vi "Disconnect source-meter(SubIV).vi"(8 "Error In":errorcluster, 11 "Loop data In":T1={"Persistent"={"Last file"=path "", "Last user"="", "Users"=[]}, "Temp handle"={"Connected"=FALSE, "Temp ctrl"={"Gain (P)"=0.0, "Reset (I)"=0.0, "Rate (D)"=0.0, "Stabilization rate"=0.0, "Stabilization delta"=0.0, "Type"=enum."Lake Shore 325", "Custom temp ctrl"={"VISA resource name"=""}, "Lakeshore 325"={"VISA name"="", "Loop"=0, "Heater Range"=1, "Heater Resistance"=0, "Sample sensor"=0, "Fast sensor"=0, "Slow sensor"=0}, "Lakeshore 331"={"VISA name"="", "Loop"=1, "Heater Range"=0, "Sample sensor"=0, "Fast sensor"=0, "Slow sensor"=0}, "Lakeshore 332"={"VISA name"="", "Loop"=1, "Heater Range"=0, "Sample sensor"=0, "Fast sensor"=0, "Slow sensor"=0}, "Lakeshore 335"={"VISA name"="", "Loop"=1, "Sample sensor"=0, "Fast sensor"=0, "Slow sensor"=0}}}, "Paths"={"Manual"=path "", "Settings"=path "", "Persistent"=path "", "Work dir."=path ""}, "Settings"={"MFIA"={"Address"="", "Use compensation"=TRUE, "Shut down gracefully"=FALSE}, "Temp ctrl"={"Gain (P)"=0.0, "Reset (I)"=0.0, "Rate (D)"=0.0, "Stabilization rate"=0.0, "Stabilization delta"=0.0, "Type"=enum."Lake Shore 325", "Custom temp ctrl"={"VISA resource name"=""}, "Lakeshore 325"={"VISA name"="", "Loop"=0, "Heater Range"=1, "Heater Resistance"=0, "Sample sensor"=0, "Fast sensor"=0, "Slow sensor"=0}, "Lakeshore 331"={"VISA name"="", "Loop"=1, "Heater Range"=0, "Sample sensor"=0, "Fast sensor"=0, "Slow sensor"=0}, "Lakeshore 332"={"VISA name"="", "Loop"=1, "Heater Range"=0, "Sample sensor"=0, "Fast sensor"=0, "Slow sensor"=0}, "Lakeshore 335"={"VISA name"="", "Loop"=1, "Sample sensor"=0, "Fast sensor"=0, "Slow sensor"=0}}, "Source-meter"={"Type"=enum."Custom", "Custom source-meter"={"VISA resource name"=""}, "Keithley 2600"={"VISA name"=""}}, "Other"={"Enable OriginLab"=FALSE, "Reader mode"=FALSE, "Auto-save"=FALSE}, "Defaults"={"IV properties"={"T"=0.0, "Vstart"=-0.5, "Vstop"=0.5, "Vpoints"=10.0, "Settling"=0.01, "I limit"=0.1, "Log mapping"=FALSE, "Averaging"=0.0}, "CV properties"={"T"=0.0, "Vstart"=-0.5, "Vstop"=0.5, "Vpoints"=10.0, "Precision"=enum."Normal", "Test signal"=0.01, "Auto I range"=FALSE, "Test frequency"=100000.0, "I range"=-2.0, "V range"=10.0, "Log mapping"=FALSE, "Rel perm"=0.0, "Area"=0.0}, "DLTS properties"={"Tstart"=0.0, "Instant start"=FALSE, "Tstop"=0.0, "T rate"=0.0, "Test signal"=0.0, "Test frequency"=0.0, "Bandwidth"=0.0, "Averaging"=0.0, "Vbias"=0.0, "Vpulse"=0.0, "pulse length"=0.0, "Pulse 2"=FALSE, "Vpulse 2"=0.0, "pulse length 2"=0.0, "I range"=-2.0, "V range"=10.0, "Emission rate"=[], "Sampling rate"=0.0, "Acq. delay"=0.0}, "LDLTS properties"={"T"=0.0, "Test signal"=0.0, "Test frequency"=0.0, "Bandwidth"=0.0, "Averaging"=0.0, "Vbias"=0.0, "Vpulse"=0.0, "pulse length"=0.0, "Pulse 2"=FALSE, "Vpulse 2"=0.0, "pulse length 2"=0.0, "I range"=-2.0, "V range"=10.0, "Sampling rate"=0.0, "Acq. delay"=0.0, "Sampling time"=0.0}}}, "Software version"=0.0, "MFIA handle"={"ziHandle"={"handleValid"=FALSE, "Conn"=0, "Path Prefix"="", "Handle"=0, "Connected"=FALSE, "Clockbase(s)"=0.0}, "Selected device"="", "ziModHandle"={"handleValid"=FALSE, "Conn"=0, "ModHandle"=0, "moduleID"="", "Path Prefix"=""}}, "Source-meter handle"={"Connected"=FALSE, "Source-meter"={"Type"=enum."Custom", "Custom source-meter"={"VISA resource name"=""}, "Keithley 2600"={"VISA name"=""}}}} {"MFIA handle"."ziModHandle"."ModHandle" format="0x%08x"; "MFIA handle"."ziModHandle"."Conn" format="0x%08x"; "MFIA handle"."ziHandle"."Handle" format="0x%08x"; "MFIA handle"."ziHandle"."Conn" format="0x%08x"; "Settings"."Defaults"."LDLTS properties"."V range" items=["10mV"=0.01, "100mV"=0.1, "1V"=1.0, "10V"=10.0]; "Settings"."Defaults"."LDLTS properties"."I range" items=["100nA"=-7.0, "1µA"=-6.0, "10µA"=-5.0, "100µA"=-4.0, "1mA"=-3.0, "10mA"=-2.0]; "Settings"."Defaults"."DLTS properties"."V range" items=["10mV"=0.01, "100mV"=0.1, "1V"=1.0, "10V"=10.0]; "Settings"."Defaults"."DLTS properties"."I range" items=["10mV"=0.01, "100mV"=0.1, "1V"=1.0, "10V"=10.0]; "Settings"."Defaults"."CV properties"."V range" items=["10mV"=0.01, "100mV"=0.1, "1V"=1.0, "10V"=10.0]; "Settings"."Defaults"."CV properties"."I range" items=["100nA"=-7.0, "1µA"=-6.0, "10µA"=-5.0, "100µA"=-4.0, "1mA"=-3.0, "10mA"=-2.0]; "Settings"."Defaults"."IV properties"."Settling" min=0.0 max=65535.0; "Settings"."Temp ctrl"."Lakeshore 335"."Slow sensor" items=["A", "B"]; "Settings"."Temp ctrl"."Lakeshore 335"."Fast sensor" items=["A", "B"]; "Settings"."Temp ctrl"."Lakeshore 335"."Sample sensor" items=["A", "B"]; "Settings"."Temp ctrl"."Lakeshore 335"."Loop" items=["Loop 1"=1, "Loop 2"=2]; "Settings"."Temp ctrl"."Lakeshore 332"."Slow sensor" items=["A", "B"]; "Settings"."Temp ctrl"."Lakeshore 332"."Fast sensor" items=["A", "B"]; "Settings"."Temp ctrl"."Lakeshore 332"."Sample sensor" items=["A", "B"]; "Settings"."Temp ctrl"."Lakeshore 332"."Heater Range" items=["Off", "Low (0.5W)", "Med (5W)", "High (50W)"]; "Settings"."Temp ctrl"."Lakeshore 332"."Loop" items=["Loop 1", "Loop 2"]; "Settings"."Temp ctrl"."Lakeshore 331"."Slow sensor" items=["A", "B"]; "Settings"."Temp ctrl"."Lakeshore 331"."Fast sensor" items=["A", "B"]; "Settings"."Temp ctrl"."Lakeshore 331"."Sample sensor" items=["A", "B"]; "Settings"."Temp ctrl"."Lakeshore 331"."Heater Range" items=["Off", "Low (0.5W)", "Med (5W)", "High (50W)"]; "Settings"."Temp ctrl"."Lakeshore 331"."Loop" items=["Loop 1", "Loop 2"]; "Settings"."Temp ctrl"."Lakeshore 325"."Slow sensor" items=["A", "B"]; "Settings"."Temp ctrl"."Lakeshore 325"."Fast sensor" items=["A", "B"]; "Settings"."Temp ctrl"."Lakeshore 325"."Sample sensor" items=["A", "B"]; "Settings"."Temp ctrl"."Lakeshore 325"."Heater Resistance" items=["25 Ohm"=1, "50 Ohm"=2]; "Settings"."Temp ctrl"."Lakeshore 325"."Heater Range" items=["Off", "Low (loop 1) or On (loop 2)", "High (loop 1)"]; "Settings"."Temp ctrl"."Lakeshore 325"."Loop" items=["Loop 1"=1, "Loop 2"=2]; "Temp handle"."Temp ctrl"."Lakeshore 335"."Slow sensor" items=["A", "B"]; "Temp handle"."Temp ctrl"."Lakeshore 335"."Fast sensor" items=["A", "B"]; "Temp handle"."Temp ctrl"."Lakeshore 335"."Sample sensor" items=["A", "B"]; "Temp handle"."Temp ctrl"."Lakeshore 335"."Loop" items=["Loop 1"=1, "Loop 2"=2]; "Temp handle"."Temp ctrl"."Lakeshore 332"."Slow sensor" items=["A", "B"]; "Temp handle"."Temp ctrl"."Lakeshore 332"."Fast sensor" items=["A", "B"]; "Temp handle"."Temp ctrl"."Lakeshore 332"."Sample sensor" items=["A", "B"]; "Temp handle"."Temp ctrl"."Lakeshore 332"."Heater Range" items=["Off", "Low (0.5W)", "Med (5W)", "High (50W)"]; "Temp handle"."Temp ctrl"."Lakeshore 332"."Loop" items=["Loop 1", "Loop 2"]; "Temp handle"."Temp ctrl"."Lakeshore 331"."Slow sensor" items=["A", "B"]; "Temp handle"."Temp ctrl"."Lakeshore 331"."Fast sensor" items=["A", "B"]; "Temp handle"."Temp ctrl"."Lakeshore 331"."Sample sensor" items=["A", "B"]; "Temp handle"."Temp ctrl"."Lakeshore 331"."Heater Range" items=["Off", "Low (0.5W)", "Med (5W)", "High (50W)"]; "Temp handle"."Temp ctrl"."Lakeshore 331"."Loop" items=["Loop 1", "Loop 2"]; "Temp handle"."Temp ctrl"."Lakeshore 325"."Slow sensor" items=["A", "B"]; "Temp handle"."Temp ctrl"."Lakeshore 325"."Fast sensor" items=["A", "B"]; "Temp handle"."Temp ctrl"."Lakeshore 325"."Sample sensor" items=["A", "B"]; "Temp handle"."Temp ctrl"."Lakeshore 325"."Heater Resistance" items=["25 Ohm"=1, "50 Ohm"=2]; "Temp handle"."Temp ctrl"."Lakeshore 325"."Heater Range" items=["Off", "Low (loop 1) or On (loop 2)", "High (loop 1)"]; "Temp handle"."Temp ctrl"."Lakeshore 325"."Loop" items=["Loop 1"=1, "Loop 2"=2]}) -> (0 "Error Out":errorcluster, 3 "Loop data Out":T1={"Persistent"={"Last file"=path "", "Last user"="", "Users"=[]}, "Temp handle"={"Connected"=FALSE, "Temp ctrl"={"Gain (P)"=0.0, "Reset (I)"=0.0, "Rate (D)"=0.0, "Stabilization rate"=0.0, "Stabilization delta"=0.0, "Type"=enum."Lake Shore 325", "Custom temp ctrl"={"VISA resource name"=""}, "Lakeshore 325"={"VISA name"="", "Loop"=0, "Heater Range"=1, "Heater Resistance"=0, "Sample sensor"=0, "Fast sensor"=0, "Slow sensor"=0}, "Lakeshore 331"={"VISA name"="", "Loop"=1, "Heater Range"=0, "Sample sensor"=0, "Fast sensor"=0, "Slow sensor"=0}, "Lakeshore 332"={"VISA name"="", "Loop"=1, "Heater Range"=0, "Sample sensor"=0, "Fast sensor"=0, "Slow sensor"=0}, "Lakeshore 335"={"VISA name"="", "Loop"=1, "Sample sensor"=0, "Fast sensor"=0, "Slow sensor"=0}}}, "Paths"={"Manual"=path "", "Settings"=path "", "Persistent"=path "", "Work dir."=path ""}, "Settings"={"MFIA"={"Address"="", "Use compensation"=TRUE, "Shut down gracefully"=FALSE}, "Temp ctrl"={"Gain (P)"=0.0, "Reset (I)"=0.0, "Rate (D)"=0.0, "Stabilization rate"=0.0, "Stabilization delta"=0.0, "Type"=enum."Lake Shore 325", "Custom temp ctrl"={"VISA resource name"=""}, "Lakeshore 325"={"VISA name"="", "Loop"=0, "Heater Range"=1, "Heater Resistance"=0, "Sample sensor"=0, "Fast sensor"=0, "Slow sensor"=0}, "Lakeshore 331"={"VISA name"="", "Loop"=1, "Heater Range"=0, "Sample sensor"=0, "Fast sensor"=0, "Slow sensor"=0}, "Lakeshore 332"={"VISA name"="", "Loop"=1, "Heater Range"=0, "Sample sensor"=0, "Fast sensor"=0, "Slow sensor"=0}, "Lakeshore 335"={"VISA name"="", "Loop"=1, "Sample sensor"=0, "Fast sensor"=0, "Slow sensor"=0}}, "Source-meter"={"Type"=enum."Custom", "Custom source-meter"={"VISA resource name"=""}, "Keithley 2600"={"VISA name"=""}}, "Other"={"Enable OriginLab"=FALSE, "Reader mode"=FALSE, "Auto-save"=FALSE}, "Defaults"={"IV properties"={"T"=0.0, "Vstart"=-0.5, "Vstop"=0.5, "Vpoints"=10.0, "Settling"=0.01, "I limit"=0.1, "Log mapping"=FALSE, "Averaging"=0.0}, "CV properties"={"T"=0.0, "Vstart"=-0.5, "Vstop"=0.5, "Vpoints"=10.0, "Precision"=enum."Normal", "Test signal"=0.01, "Auto I range"=FALSE, "Test frequency"=100000.0, "I range"=-2.0, "V range"=10.0, "Log mapping"=FALSE, "Rel perm"=0.0, "Area"=0.0}, "DLTS properties"={"Tstart"=0.0, "Instant start"=FALSE, "Tstop"=0.0, "T rate"=0.0, "Test signal"=0.0, "Test frequency"=0.0, "Bandwidth"=0.0, "Averaging"=0.0, "Vbias"=0.0, "Vpulse"=0.0, "pulse length"=0.0, "Pulse 2"=FALSE, "Vpulse 2"=0.0, "pulse length 2"=0.0, "I range"=-2.0, "V range"=10.0, "Emission rate"=[], "Sampling rate"=0.0, "Acq. delay"=0.0}, "LDLTS properties"={"T"=0.0, "Test signal"=0.0, "Test frequency"=0.0, "Bandwidth"=0.0, "Averaging"=0.0, "Vbias"=0.0, "Vpulse"=0.0, "pulse length"=0.0, "Pulse 2"=FALSE, "Vpulse 2"=0.0, "pulse length 2"=0.0, "I range"=-2.0, "V range"=10.0, "Sampling rate"=0.0, "Acq. delay"=0.0, "Sampling time"=0.0}}}, "Software version"=0.0, "MFIA handle"={"ziHandle"={"handleValid"=FALSE, "Conn"=0, "Path Prefix"="", "Handle"=0, "Connected"=FALSE, "Clockbase(s)"=0.0}, "Selected device"="", "ziModHandle"={"handleValid"=FALSE, "Conn"=0, "ModHandle"=0, "moduleID"="", "Path Prefix"=""}}, "Source-meter handle"={"Connected"=FALSE, "Source-meter"={"Type"=enum."Custom", "Custom source-meter"={"VISA resource name"=""}, "Keithley 2600"={"VISA name"=""}}}} {"MFIA handle"."ziModHandle"."ModHandle" format="0x%08x"; "MFIA handle"."ziModHandle"."Conn" format="0x%08x"; "MFIA handle"."ziHandle"."Handle" format="0x%08x"; "MFIA handle"."ziHandle"."Conn" format="0x%08x"; "Settings"."Defaults"."LDLTS properties"."V range" items=["10mV"=0.01, "100mV"=0.1, "1V"=1.0, "10V"=10.0]; "Settings"."Defaults"."LDLTS properties"."I range" items=["100nA"=-7.0, "1µA"=-6.0, "10µA"=-5.0, "100µA"=-4.0, "1mA"=-3.0, "10mA"=-2.0]; "Settings"."Defaults"."DLTS properties"."V range" items=["10mV"=0.01, "100mV"=0.1, "1V"=1.0, "10V"=10.0]; "Settings"."Defaults"."DLTS properties"."I range" items=["10mV"=0.01, "100mV"=0.1, "1V"=1.0, "10V"=10.0]; "Settings"."Defaults"."CV properties"."V range" items=["10mV"=0.01, "100mV"=0.1, "1V"=1.0, "10V"=10.0]; "Settings"."Defaults"."CV properties"."I range" items=["100nA"=-7.0, "1µA"=-6.0, "10µA"=-5.0, "100µA"=-4.0, "1mA"=-3.0, "10mA"=-2.0]; "Settings"."Defaults"."IV properties"."Settling" min=0.0 max=65535.0; "Settings"."Temp ctrl"."Lakeshore 335"."Slow sensor" items=["A", "B"]; "Settings"."Temp ctrl"."Lakeshore 335"."Fast sensor" items=["A", "B"]; "Settings"."Temp ctrl"."Lakeshore 335"."Sample sensor" items=["A", "B"]; "Settings"."Temp ctrl"."Lakeshore 335"."Loop" items=["Loop 1"=1, "Loop 2"=2]; "Settings"."Temp ctrl"."Lakeshore 332"."Slow sensor" items=["A", "B"]; "Settings"."Temp ctrl"."Lakeshore 332"."Fast sensor" items=["A", "B"]; "Settings"."Temp ctrl"."Lakeshore 332"."Sample sensor" items=["A", "B"]; "Settings"."Temp ctrl"."Lakeshore 332"."Heater Range" items=["Off", "Low (0.5W)", "Med (5W)", "High (50W)"]; "Settings"."Temp ctrl"."Lakeshore 332"."Loop" items=["Loop 1", "Loop 2"]; "Settings"."Temp ctrl"."Lakeshore 331"."Slow sensor" items=["A", "B"]; "Settings"."Temp ctrl"."Lakeshore 331"."Fast sensor" items=["A", "B"]; "Settings"."Temp ctrl"."Lakeshore 331"."Sample sensor" items=["A", "B"]; "Settings"."Temp ctrl"."Lakeshore 331"."Heater Range" items=["Off", "Low (0.5W)", "Med (5W)", "High (50W)"]; "Settings"."Temp ctrl"."Lakeshore 331"."Loop" items=["Loop 1", "Loop 2"]; "Settings"."Temp ctrl"."Lakeshore 325"."Slow sensor" items=["A", "B"]; "Settings"."Temp ctrl"."Lakeshore 325"."Fast sensor" items=["A", "B"]; "Settings"."Temp ctrl"."Lakeshore 325"."Sample sensor" items=["A", "B"]; "Settings"."Temp ctrl"."Lakeshore 325"."Heater Resistance" items=["25 Ohm"=1, "50 Ohm"=2]; "Settings"."Temp ctrl"."Lakeshore 325"."Heater Range" items=["Off", "Low (loop 1) or On (loop 2)", "High (loop 1)"]; "Settings"."Temp ctrl"."Lakeshore 325"."Loop" items=["Loop 1"=1, "Loop 2"=2]; "Temp handle"."Temp ctrl"."Lakeshore 335"."Slow sensor" items=["A", "B"]; "Temp handle"."Temp ctrl"."Lakeshore 335"."Fast sensor" items=["A", "B"]; "Temp handle"."Temp ctrl"."Lakeshore 335"."Sample sensor" items=["A", "B"]; "Temp handle"."Temp ctrl"."Lakeshore 335"."Loop" items=["Loop 1"=1, "Loop 2"=2]; "Temp handle"."Temp ctrl"."Lakeshore 332"."Slow sensor" items=["A", "B"]; "Temp handle"."Temp ctrl"."Lakeshore 332"."Fast sensor" items=["A", "B"]; "Temp handle"."Temp ctrl"."Lakeshore 332"."Sample sensor" items=["A", "B"]; "Temp handle"."Temp ctrl"."Lakeshore 332"."Heater Range" items=["Off", "Low (0.5W)", "Med (5W)", "High (50W)"]; "Temp handle"."Temp ctrl"."Lakeshore 332"."Loop" items=["Loop 1", "Loop 2"]; "Temp handle"."Temp ctrl"."Lakeshore 331"."Slow sensor" items=["A", "B"]; "Temp handle"."Temp ctrl"."Lakeshore 331"."Fast sensor" items=["A", "B"]; "Temp handle"."Temp ctrl"."Lakeshore 331"."Sample sensor" items=["A", "B"]; "Temp handle"."Temp ctrl"."Lakeshore 331"."Heater Range" items=["Off", "Low (0.5W)", "Med (5W)", "High (50W)"]; "Temp handle"."Temp ctrl"."Lakeshore 331"."Loop" items=["Loop 1", "Loop 2"]; "Temp handle"."Temp ctrl"."Lakeshore 325"."Slow sensor" items=["A", "B"]; "Temp handle"."Temp ctrl"."Lakeshore 325"."Fast sensor" items=["A", "B"]; "Temp handle"."Temp ctrl"."Lakeshore 325"."Sample sensor" items=["A", "B"]; "Temp handle"."Temp ctrl"."Lakeshore 325"."Heater Resistance" items=["25 Ohm"=1, "50 Ohm"=2]; "Temp handle"."Temp ctrl"."Lakeshore 325"."Heater Range" items=["Off", "Low (loop 1) or On (loop 2)", "High (loop 1)"]; "Temp handle"."Temp ctrl"."Lakeshore 325"."Loop" items=["Loop 1"=1, "Loop 2"=2]})   [LabVIEW 2019]
doc: "Terminates connection with source meter"
uses:
  Type defs/Loop data Type Def.ctl
  Type defs/Persistent Type Def.ctl
  Type defs/Temp handle Type Def.ctl
  Type defs/Temp ctrl Type Def.ctl
  Custom devices/Custom temp ctrl settings.ctl
  Type defs/Paths Type Def.ctl
  Type defs/Settings Type Def.ctl
  Type defs/Imps Type Def.ctl
  Type defs/Source-meter Type Def.ctl
  Custom devices/Custom source-meter settings.ctl
  Type defs/Other settings Type Def.ctl
  Type defs/IV properties Type Def.ctl
  Type defs/CV properties Type Def.ctl
  Type defs/DLTS properties Type Def.ctl
  Type defs/LDLTS properties Type Def.ctl
  Type defs/MFIA handle Type Def.ctl
  <instrlib>/Zurich Instruments LabOne/Public/ziTypeHandle.ctl
  <instrlib>/Zurich Instruments LabOne/Public/Modules/ziTypeModHandle.ctl
  Type defs/Source-meter handle Type Def.ctl
  <instrlib>/Keithley 2600 Series/Keithley 2600 Series.lvlib
  <instrlib>/Zurich Instruments LabOne/Zurich Instruments LabOne.lvlib
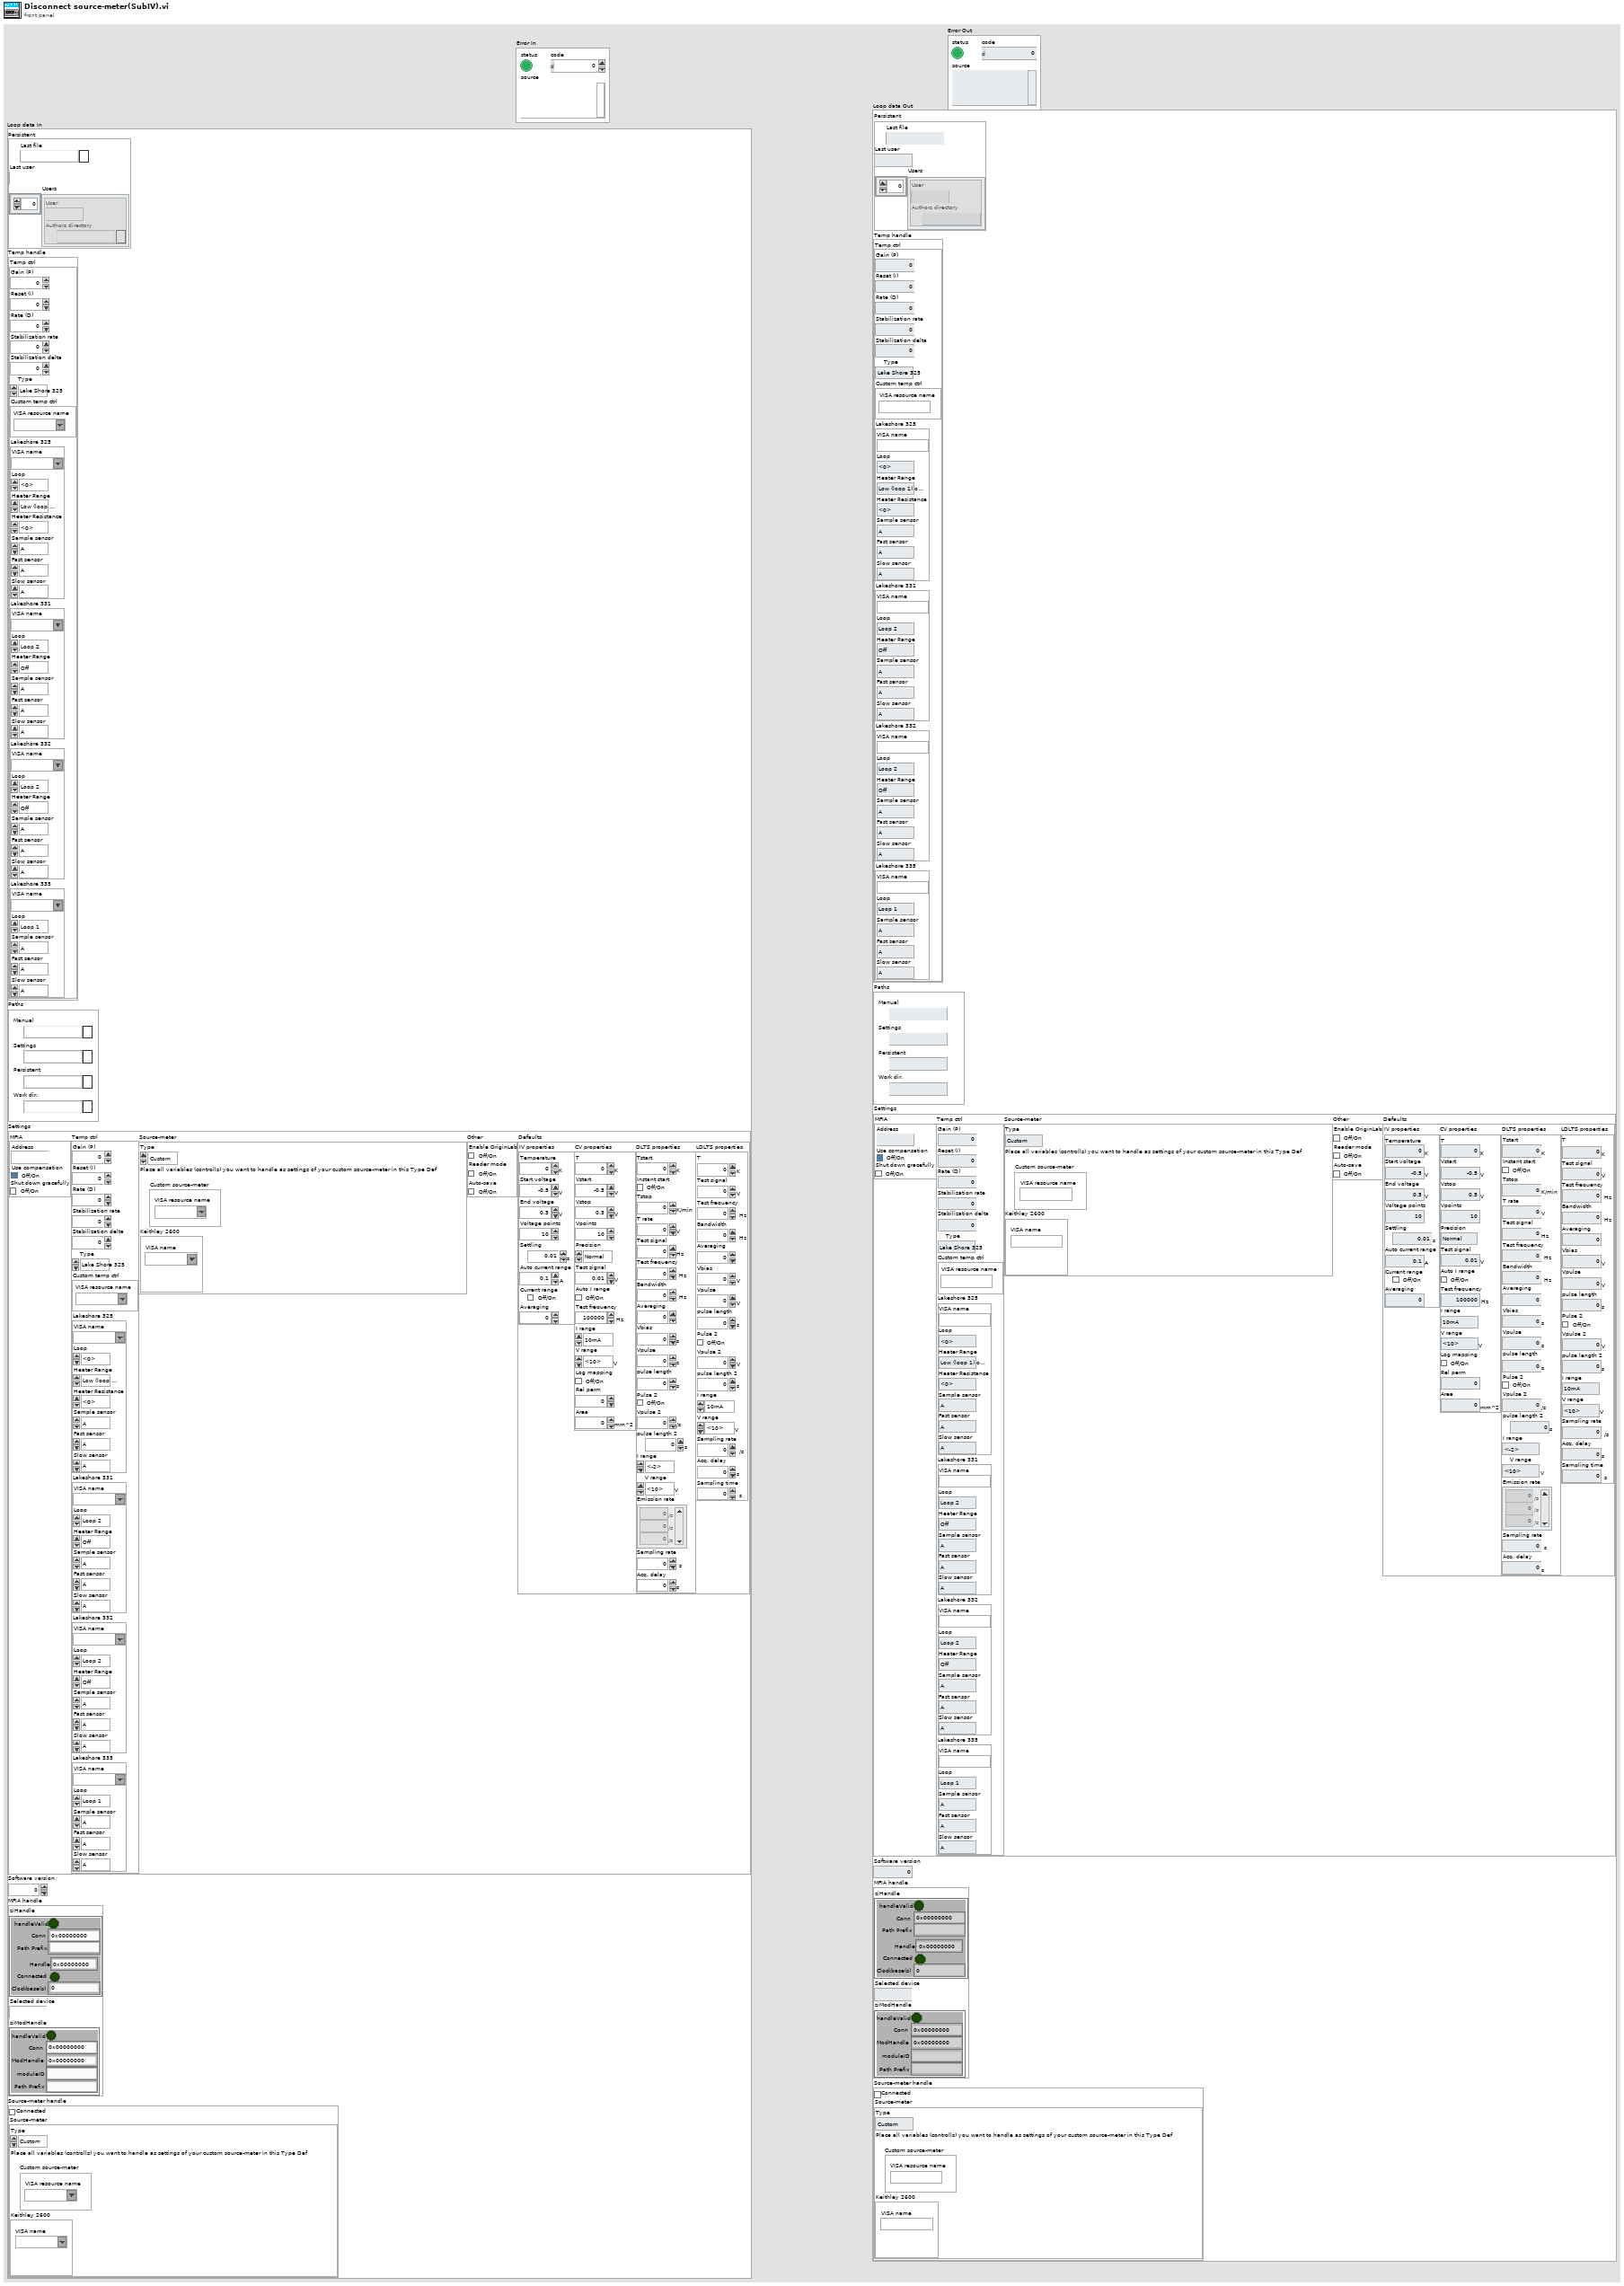
[diagram p1: front panel]
types:
  T1 = typedef "Loop data Type Def.ctl" = cluster{"Persistent":T2, "Temp handle":T3, "Paths":T6, "Settings":T7, "Software version":dbl, "MFIA handle":T16, "Source-meter handle":T19}
  T2 = typedef "Persistent Type Def.ctl" = cluster{"Last file":path, "Last user":string, "Users":cluster{"User":string, "Authors directory":path}[]}
  T3 = typedef "Temp handle Type Def.ctl" = cluster{"Connected":bool, "Temp ctrl":T4}
  T4 = typedef "Temp ctrl Type Def.ctl" = cluster{"Gain (P)":dbl, "Reset (I)":dbl, "Rate (D)":dbl, "Stabilization rate":dbl, "Stabilization delta":dbl, "Type":enum16{"Custom", "Lake Shore 325", "Lake Shore 331", "Lake Shore 332", "Lake Shore 335"}, "Custom temp ctrl":T5, "Lakeshore 325":cluster{"VISA name":refnum<visa-resource-name>, "Loop":u16, "Heater Range":u16, "Heater Resistance":u16, "Sample sensor":u16, "Fast sensor":u16, "Slow sensor":u16}, "Lakeshore 331":cluster{"VISA name":refnum<visa-resource-name>, "Loop":u16, "Heater Range":u16, "Sample sensor":u16, "Fast sensor":u16, "Slow sensor":u16}, "Lakeshore 332":cluster{"VISA name":refnum<visa-resource-name>, "Loop":u16, "Heater Range":u16, "Sample sensor":u16, "Fast sensor":u16, "Slow sensor":u16}, "Lakeshore 335":cluster{"VISA name":refnum<visa-resource-name>, "Loop":u16, "Sample sensor":u16, "Fast sensor":u16, "Slow sensor":u16}}
  T5 = typedef "Custom temp ctrl settings.ctl" = cluster{"VISA resource name":refnum<visa-resource-name>}
  T6 = typedef "Paths Type Def.ctl" = cluster{"Manual":path, "Settings":path, "Persistent":path, "Work dir.":path}
  T7 = typedef "Settings Type Def.ctl" = cluster{"MFIA":T8, "Temp ctrl":T4, "Source-meter":T9, "Other":T11, "Defaults":cluster{"IV properties":T12, "CV properties":T13, "DLTS properties":T14, "LDLTS properties":T15}}
  T8 = typedef "Imps Type Def.ctl" = cluster{"Address":string, "Use compensation":bool, "Shut down gracefully":bool}
  T9 = typedef "Source-meter Type Def.ctl" = cluster{"Type":enum16{"Custom", "Keithley 2600"}, "Custom source-meter":T10, "Keithley 2600":cluster{"VISA name":refnum<visa-resource-name>}}
  T10 = typedef "Custom source-meter settings.ctl" = cluster{"VISA resource name":refnum<visa-resource-name>}
  T11 = typedef "Other settings Type Def.ctl" = cluster{"Enable OriginLab":bool, "Reader mode":bool, "Auto-save":bool}
  T12 = typedef "IV properties Type Def.ctl" = cluster{"T":dbl[unit], "Vstart":dbl[unit], "Vstop":dbl[unit], "Vpoints":dbl, "Settling":dbl[unit], "I limit":dbl[unit], "Log mapping":bool, "Averaging":dbl}
  T13 = typedef "CV properties Type Def.ctl" = cluster{"T":dbl[unit], "Vstart":dbl[unit], "Vstop":dbl[unit], "Vpoints":dbl, "Precision":enum16{"Low (Fast)", "Normal", "High (Slow)"}, "Test signal":dbl[unit], "Auto I range":bool, "Test frequency":dbl[unit], "I range":dbl, "V range":dbl[unit], "Log mapping":bool, "Rel perm":dbl, "Area":dbl[unit]}
  T14 = typedef "DLTS properties Type Def.ctl" = cluster{"Tstart":dbl[unit], "Instant start":bool, "Tstop":dbl[unit], "T rate":dbl[unit], "Test signal":dbl[unit], "Test frequency":dbl[unit], "Bandwidth":dbl[unit], "Averaging":dbl, "Vbias":dbl[unit], "Vpulse":dbl[unit], "pulse length":dbl[unit], "Pulse 2":bool, "Vpulse 2":dbl[unit], "pulse length 2":dbl[unit], "I range":dbl, "V range":dbl[unit], "Emission rate":dbl[unit][], "Sampling rate":dbl[unit], "Acq. delay":dbl[unit]}
  T15 = typedef "LDLTS properties Type Def.ctl" = cluster{"T":dbl[unit], "Test signal":dbl[unit], "Test frequency":dbl[unit], "Bandwidth":dbl[unit], "Averaging":dbl, "Vbias":dbl[unit], "Vpulse":dbl[unit], "pulse length":dbl[unit], "Pulse 2":bool, "Vpulse 2":dbl[unit], "pulse length 2":dbl[unit], "I range":dbl, "V range":dbl[unit], "Sampling rate":dbl[unit], "Acq. delay":dbl[unit], "Sampling time":dbl[unit]}
  T16 = typedef "MFIA handle Type Def.ctl" = cluster{"ziHandle":T17, "Selected device":string, "ziModHandle":T18}
  T17 = typedef "Zurich Instruments LabOne.lvlib/ziTypeHandle.ctl" = cluster{"handleValid":bool, "Conn":u64, "Path Prefix":string, "Handle":u64, "Connected":bool, "Clockbase(s)":dbl}
  T18 = typedef "Zurich Instruments LabOne.lvlib/ziTypeModHandle.ctl" = cluster{"handleValid":bool, "Conn":u64, "ModHandle":u64, "moduleID":string, "Path Prefix":string}
  T19 = typedef "Source-meter handle Type Def.ctl" = cluster{"Connected":bool, "Source-meter":T9}
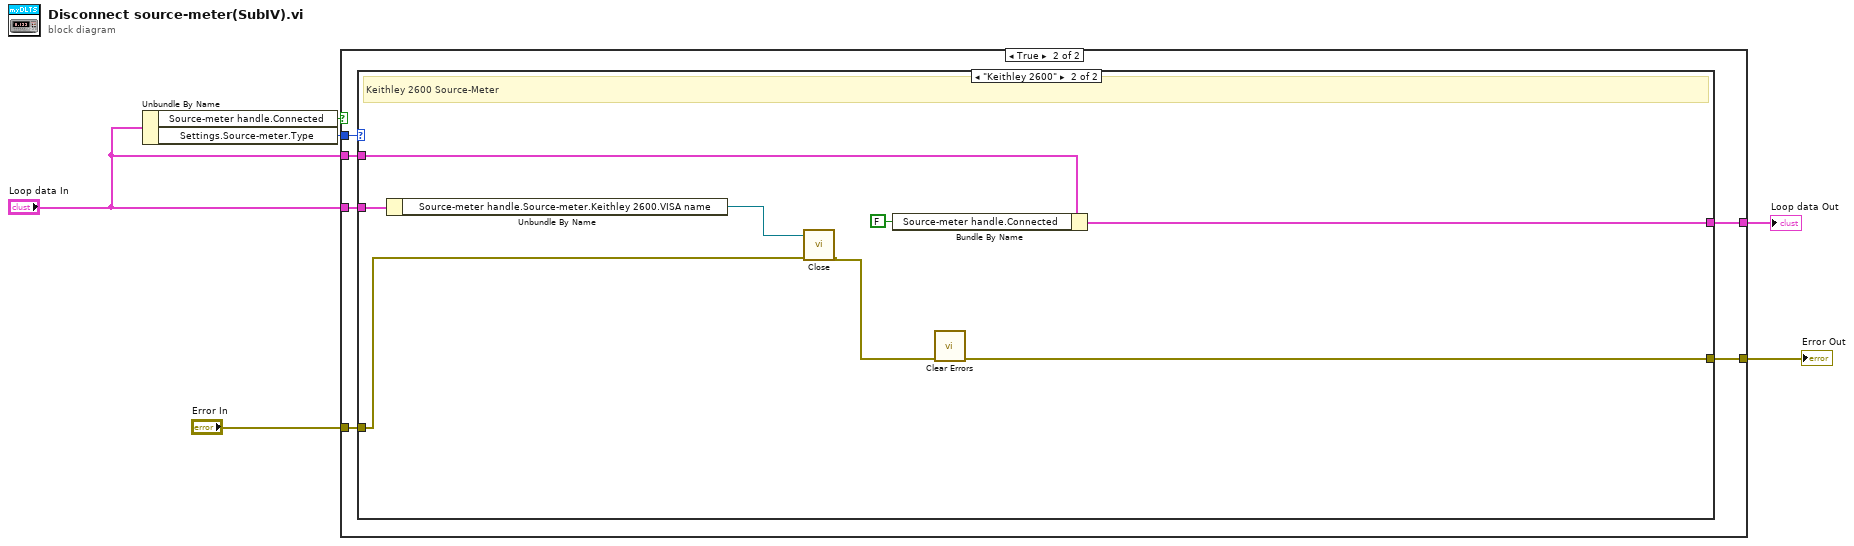
[diagram p0: block diagram]
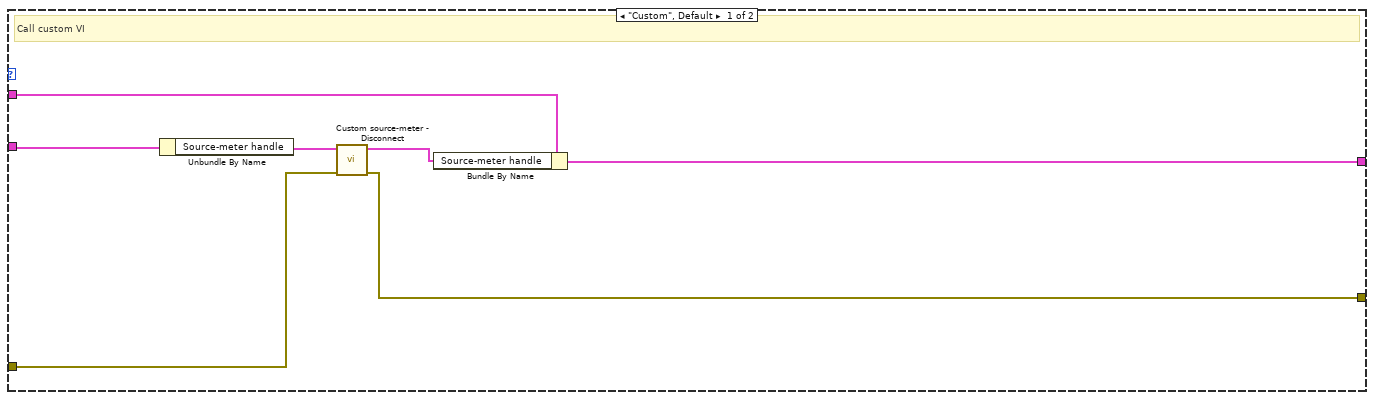
[diagram p3: hidden frame]
diagram:
  n1 = Unbundle By Name("Loop data In") -> ("Source-meter handle.Connected"=w3:bool, "Settings.Source-meter.Type"=w2:enum16{"Custom", "Keithley 2600"})
  n2 = case shown="True" w3 {
    tunnel: [w8 w14] -> w6
    tunnel: "Error In" -> [w7 w13]
    tunnel: "Loop data In" -> [w8 w12]
    tunnel: [w7 w11] -> w4
    tunnel: w2 -> [_ w10]
    tunnel: "Loop data In" -> [_ w9]
    frame False {
      # "Controller is already disconnected"
    }
    frame True {
      n3 = case shown="\"Keithley 2600\"" w10 {
        tunnel: [w19 w25] -> w14
        tunnel: w13 -> [w16 w23]
        tunnel: w12 -> [w20 w27]
        tunnel: [w15 w28] -> w11
        tunnel: w9 -> [w21 w29]
        frame "Custom", Default {
          # "Call custom VI"
          n4 = Unbundle By Name(w21) -> ("Source-meter handle"=w18:T19)
          n5 = call "Custom source-meter - Disconnect.vi"("Error In"=w16, "Source-meter handle in"=w18) -> ("Error Out"=w15:errorcluster, "Source-meter handle out"=w17:T19)  [unwired: 8 in]
          n6 = Bundle By Name(cluster=w20, "Source-meter handle"=w17) -> (w19:T1)
        }
        frame "Keithley 2600" {
          # "Keithley 2600 Source-Meter"
          n7 = Unbundle By Name(w29) -> ("Source-meter handle.Source-meter.Keithley 2600.VISA name"=w24:refnum<visa-resource-name>)
          n8 = call <instrlib>:"Close.vi"("error in (no error)"=w23, "VISA resource name"=w24) -> ("error out"=w22:errorcluster)  [unwired: 9 in]
          n9 = Bundle By Name(cluster=w27, "Source-meter handle.Connected"=FALSE ("Temp handle.Connected")) -> (w25:T1)
          n10 = call <vilib>:"Clear Errors.vi"("error in (no error)"=w22) -> ("error out"=w28:errorcluster)  [unwired: 5 in, 1 out]
        }
      }
    }
  }
  "Loop data Out" <- w6
  "Error Out" <- w4
